vi "fgv_agv_status_data.vi"(7 "cmd":T4, 8 "error in":errorcluster, 9 "Light status in":T1, 10 "Motor status in":T2, 11 "AGV status in":T3={"System Feedback"={"system state"="normal", "Control Mode"=0, "Battery Voltage (V)"=27.3, "error code High"=0, "error code Low"=0}, "Motion Feedback"={"Linear Velocity (m/s)"=-0.982, "Angular Velocity (rad/s)"=-0.008}} {"Motion Feedback"."Linear Velocity (m/s)" format="%.2f"; "Motion Feedback"."Angular Velocity (rad/s)" format="%.2f"}) -> (0 "error out":errorcluster, 1 "Light Feedback out":T1, 2 "Motor status out":T2, 3 "AGV status info out":T3={"System Feedback"={"system state"="normal", "Control Mode"=0, "Battery Voltage (V)"=27.3, "error code High"=0, "error code Low"=0}, "Motion Feedback"={"Linear Velocity (m/s)"=-0.982, "Angular Velocity (rad/s)"=-0.008}} {"Motion Feedback"."Linear Velocity (m/s)" format="%.2f"; "Motion Feedback"."Angular Velocity (rad/s)" format="%.2f"})   [LabVIEW 2019]
uses:
  Ctrl/agv_status.ctl
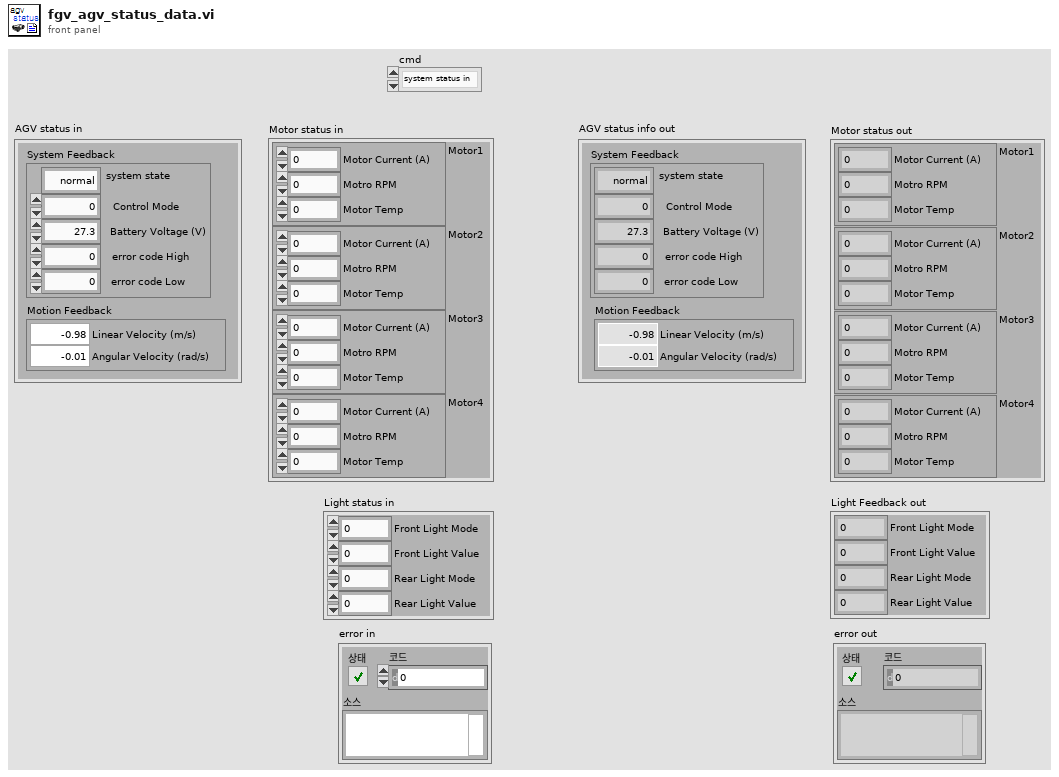
[diagram p1: front panel]
types:
  T1 = cluster{"Front Light Mode":i8, "Front Light Value":i8, "Rear Light Mode":i8, "Rear Light Value":i8}
  T2 = cluster{"Motor1":cluster{"Motor Current (A)":dbl, "Motro RPM":u16, "Motor Temp":i8}, "Motor2":cluster{"Motor Current (A)":dbl, "Motro RPM":u16, "Motor Temp":i8}, "Motor3":cluster{"Motor Current (A)":dbl, "Motro RPM":u16, "Motor Temp":i8}, "Motor4":cluster{"Motor Current (A)":dbl, "Motro RPM":u16, "Motor Temp":i8}}
  T3 = cluster{"System Feedback":cluster{"system state":string, "Control Mode":u8, "Battery Voltage (V)":dbl, "error code High":u8, "error code Low":u8}, "Motion Feedback":cluster{"Linear Velocity (m/s)":dbl, "Angular Velocity (rad/s)":dbl}}
  T4 = typedef "agv_status.ctl" = enum16{"system status in", "motor status in", "light status in", "read"}
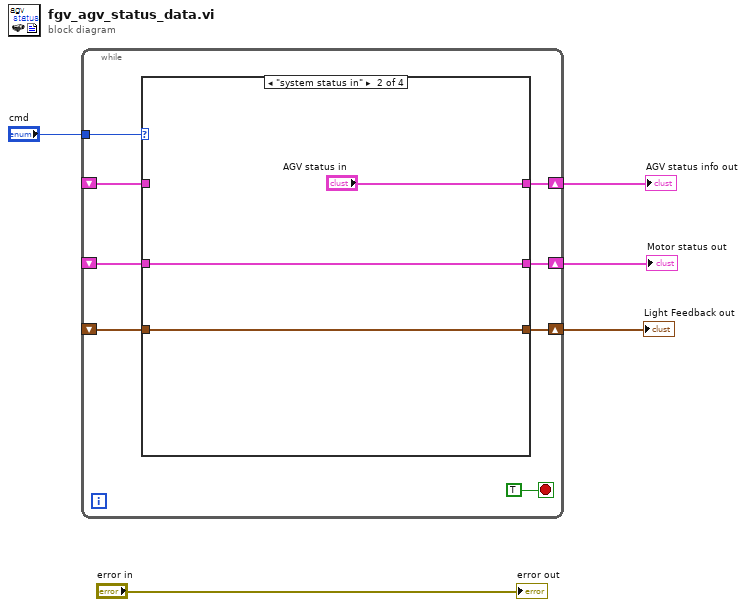
[diagram p0: block diagram]
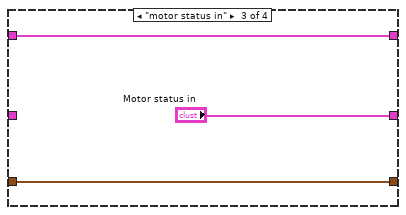
[diagram p3: hidden frame]
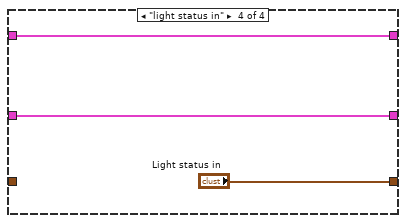
[diagram p4: hidden frame]
diagram:
  n1 = while {
    tunnel: "cmd" -> [w12]
    shift-right: [w11] -> w4
    shift-left: _ -> [w10]
    shift-right: [w9] -> w3
    shift-left: _ -> [w8]
    shift-right: [w7] -> w2
    shift-left: _ -> [w6]
    stop <- TRUE stop-if-true
    n2 = case shown="\"system status in\"" w12 {
      tunnel: [w16 "AGV status in" w21 w23] -> w11
      tunnel: w10 -> [w16 _ w21 w23]
      tunnel: [w15 w18 "Motor status in" w24] -> w9
      tunnel: w8 -> [w15 w18 _ w24]
      tunnel: [w14 w17 w20 "Light status in"] -> w7
      tunnel: w6 -> [w14 w17 w20 _]
      frame "read", Default {
      }
      frame "system status in" {
      }
      frame "motor status in" {
      }
      frame "light status in" {
      }
    }
  }
  "AGV status info out" <- w4
  "Light Feedback out" <- w2
  "Motor status out" <- w3
  "error out" <- "error in"
